vi "update states from tdms.vi"(8 "error in (no error)":errorcluster, 10 "output cluster":T1, 11 "5785_3.2GHz_one channel in":refnum<class "5785_3.2GHz_one channel.lvclass">) -> (0 "error out":errorcluster, 2 "tdms file mode":T2=enum."P2P - VST", 3 "5785_3.2GHz_one channel out":refnum<class "5785_3.2GHz_one channel.lvclass">)   [LabVIEW 2021, in "5785_3.2GHz_one channel.lvclass"]
uses:
  5785_3.2GHz_one channel.lvclass
  pulse_tx_vis/CTL/device_mode.ctl
  device_type/device_type.lvclass
  5785_3.2GHz_one channel.lvclass/5785_3.2GHz_one channel.ctl
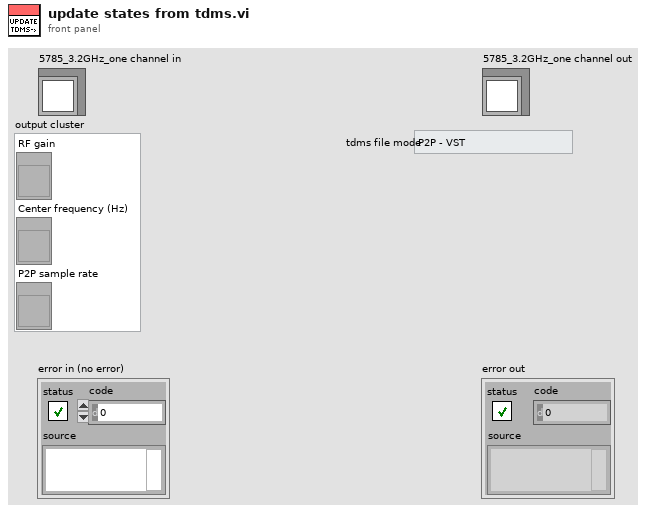
[diagram p1: front panel]
types:
  T1 = cluster{"RF gain ":refnum<vi>, "Center frequency (Hz) ":refnum<vi>, "P2P sample rate":refnum<vi>}
  T2 = typedef "device_mode.ctl" = enum16{"USRP - 180MHz", "5785 - 2*180MHz", "5785 - 3.2GHz", "P2P - VST", "5785 2*1.6GHz"}
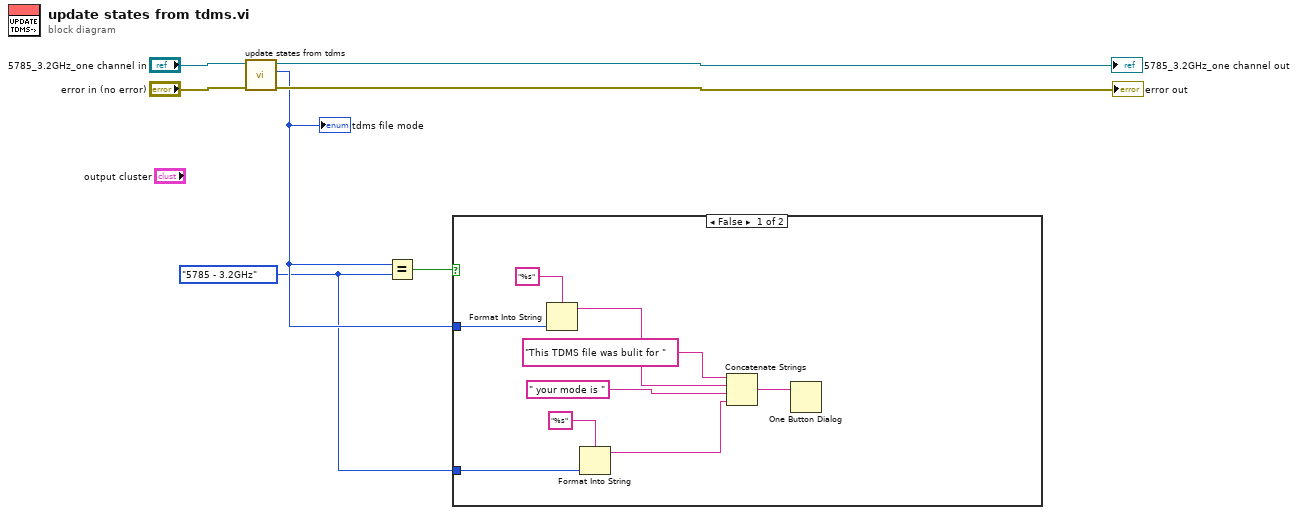
[diagram p0: block diagram]
diagram:
  w1 = device_mode."5785 - 3.2GHz" ("Mode")
  n1 = call-parent "update states from tdms.vi"("error in (no error)"="error in (no error)", "device_type in"="5785_3.2GHz_one channel in") -> ("error out"=→"error out":errorcluster, "tdms file mode"=w2:T2, "device_type out"=→"5785_3.2GHz_one channel out":refnum<class "5785_3.2GHz_one channel.lvclass">)  [unwired: 7 in]
  "tdms file mode" <- w2
  n2 = Equal?(x=w2, y=w1) -> (x = y?=w3:bool)
  n3 = case shown="False" w3 {
    tunnel: w2 -> [w15 _]
    tunnel: w1 -> [w10 _]
    frame False {
      n4 = Format Into String(format string="%s", w15) -> (resulting string=w14:string)  [unwired: 2 in, 1 out]
      n5 = Format Into String(format string="%s", w10) -> (resulting string=w9:string)  [unwired: 2 in, 1 out]
      n6 = Concatenate Strings("This TDMS file was bulit for " ("string"), w14, " your mode is " ("string"), w9) -> (w8:string)
      n7 = One Button Dialog(message=w8) -> ()  [unwired: 1 in, 1 out]
    }
    frame True {
    }
  }
